vi "AI_ReadScaledData.vi"(3 "error in (no error)":errorcluster, 4 "count":i32, 6 "Task ID":u32) -> (0 "error out":errorcluster, 1 "data":dbl[](array[numeric]), 2 "Task ID":u32)   [LabVIEW 2015]
uses:
  Windows/System32/AdvLvDaq.dll
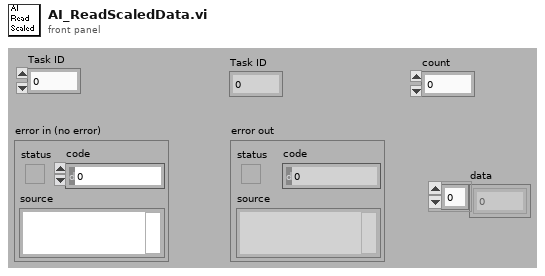
[diagram p1: front panel]
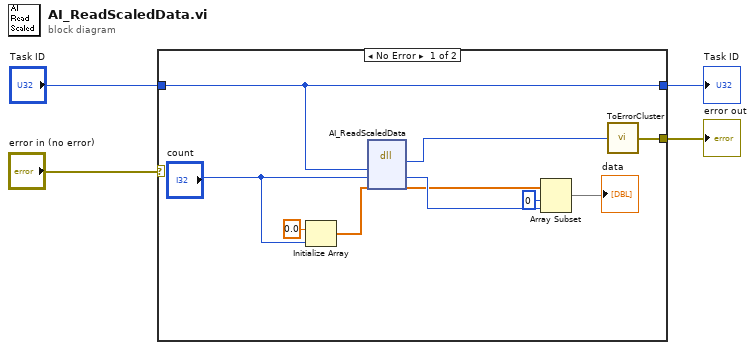
[diagram p0: block diagram]
diagram:
  n1 = case shown="No Error" "error in (no error)" {
    selector: "error in (no error)" -> [_ w16]
    tunnel: "Task ID" -> [w12 w15]
    tunnel: [w13 w16] -> w2
    tunnel: [w12 w15] -> w1
    frame No Error {
      n2 = Initialize Array(0.0 ("element"), "count") -> (w10:dbl[])
      n3 = dll-call lib="C:/Windows/System32/AdvLvDaq.dll" fn="AI_ReadScaledData"("taskId"=w12, "count"="count", "data"=w10) -> ("return type"=w14:i32, "count"=w7:i32, "data"=w6:dbl[])  [unwired: 4 in, 2 out]
      n4 = Array Subset(array=w6, index=0, length=w7) -> (→"data":dbl[])
      n5 = call "ToErrorCluster.vi"("error code"=w14) -> ("error out"=w13:errorcluster)
    }
    frame Error {
    }
  }
  "error out" <- w2
  "Task ID" <- w1
